vi "Funcion_Escribir_B.vi"(8 "Array":bool[](array[boolean]), 9 "PIPES ENTRADA":cluster{"PIPE_IN":i32, "PIPE_OUT":i32}, 11 "error in (no error)":errorcluster) -> (1 "PIPES SALIDA":cluster{"PIPE_IN":i32, "PIPE_OUT":i32}, 3 "error out":errorcluster)   [LabVIEW 2016]
uses:
  microchip_solutions_v2013-06-15/USB/Tools/MCHPUSB Custom Driver/Mpusbapi/Dll/Borland_C/mpusbapi.dll
panel:
  out "pLength":i32
  out "string":string
  out "number":u32
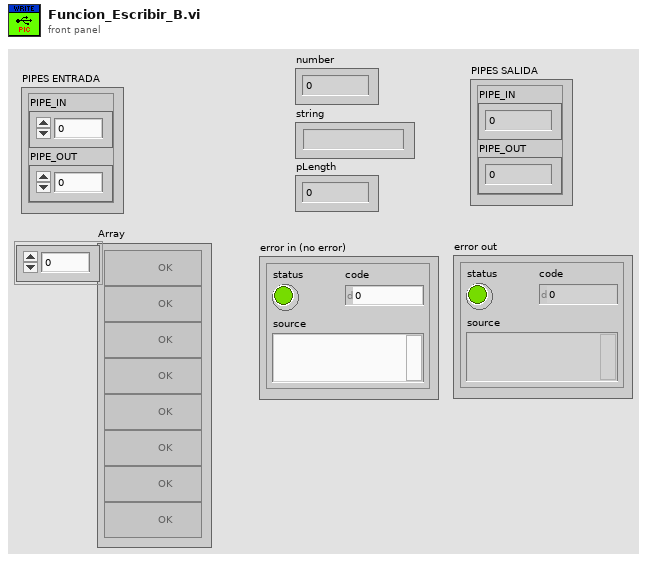
[diagram p1: front panel]
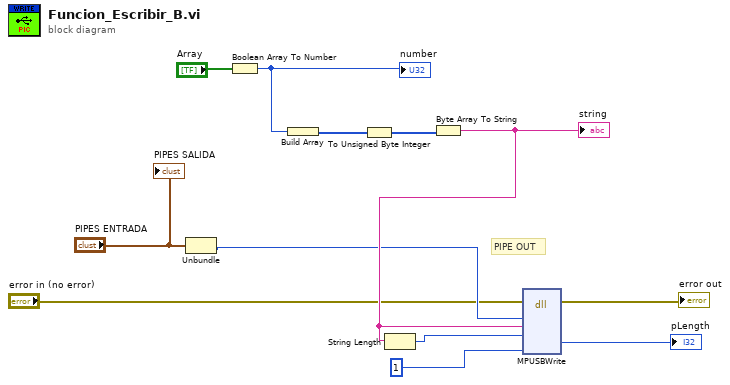
[diagram p0: block diagram]
diagram:
  # "PIPE OUT"
  n1 = Unbundle("PIPES ENTRADA") -> ("PIPE_OUT"=w3:i32)  [unwired: 1 out]
  n2 = Boolean Array To Number(Boolean array="Array") -> (number=w10:u32)
  "number" <- w10
  n3 = Build Array "Build Array"(w10) -> (w11:u32[])
  n4 = To Unsigned Byte Integer(number=w11) -> (unsigned 8bit integer=w9:u8[])
  n5 = Byte Array To String(unsigned byte array=w9) -> (string=w8:string)
  "string" <- w8
  n6 = String Length(string=w8) -> (length=w7:i32)
  n7 = dll-call lib="C:/microchip_solutions_v2013-06-15/USB/Tools/MCHPUSB Custom Driver/Mpusbapi/Dll/Borland_C/mpusbapi.dll" fn="MPUSBWrite"(error in="error in (no error)", "PIPE OUT"=w3, "pData"=w8, "dwLength"=w7, "Milliseconds"=1) -> (error out=→"error out":errorcluster, "pLength"=→"pLength":i32)  [unwired: 8 in, 1 out]
  "PIPES SALIDA" <- "PIPES ENTRADA"
